vi "general.errorDialog.vi"(7 "error in":bool, 10 "Response":string, 11 "Original command":string) -> (3 "out":bool)   [LabVIEW 2011]
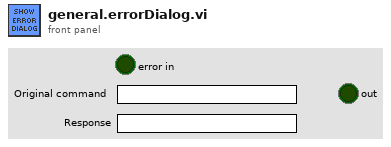
[diagram p1: front panel]
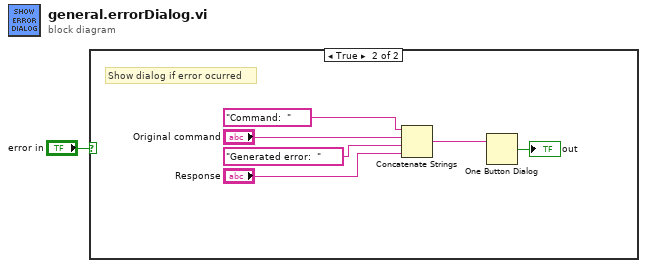
[diagram p0: block diagram]
diagram:
  n1 = case shown="True" "error in" {
    frame False {
      # "No error happenend"
    }
    frame True {
      # "Show dialog if error ocurred"
      n2 = Concatenate Strings("Command:  ", "Original command", "Generated error:  ", "Response") -> (w3:string)
      n3 = One Button Dialog(message=w3) -> (true=→"out":bool)  [unwired: 1 in]
    }
  }
